vi "Clear Reservation.vi"(0 "reference in":refnum<class "Simulated-PowerModule.lvclass">, 11 "Error In":errorcluster) -> (4 "reference out":refnum<class "Simulated-PowerModule.lvclass">, 15 "Error Out":errorcluster)   [LabVIEW 2023, in "Simulated-PowerModule.lvlib" / "Simulated-PowerModule.lvclass"]
uses:
  Simulated-PowerModule.lvclass
  Simulated-PowerModule.lvclass/Simulated-PowerModule.ctl
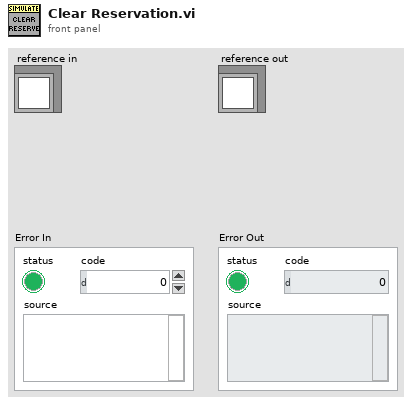
[diagram p1: front panel]
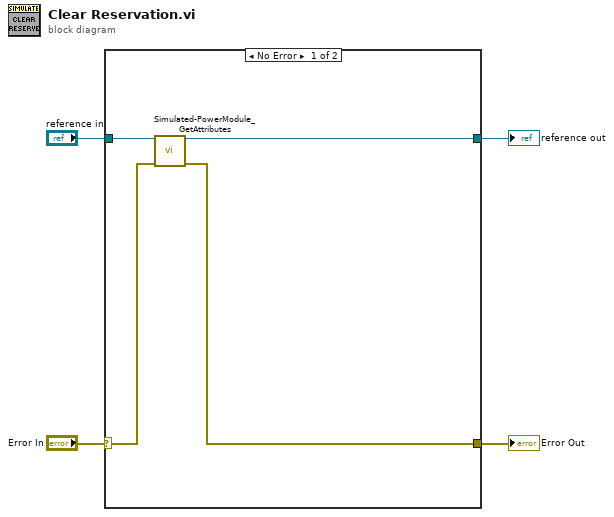
[diagram p0: block diagram]
diagram:
  n1 = case shown="No Error" "Error In" {
    selector: "Error In" -> [w7 w9]
    tunnel: "reference in" -> [w8 w10]
    tunnel: [w6 w10] -> w4
    tunnel: [w5 w9] -> w3
    frame No Error {
      n2 = call "Simulated-PowerModule_GetAttributes.vi"("reference in"=w8, "Error In"=w7) -> ("reference out"=w6:refnum<class "Simulated-PowerModule.lvclass">, "Error Out"=w5:errorcluster)  [unwired: 10 in, 2 out]
    }
    frame Error {
    }
  }
  "Error Out" <- w3
  "reference out" <- w4
